vi "Sub00_Setup.vi"(7 "Enum":T1(ring), 8 "error in (no error)":errorcluster, 9 "Tab Control":T2(tab), 10 "Select sequence":string(combo)="F1", 11 "Path":path) -> (0 "error out":errorcluster, 1 "filenames":string[](array[string]), 2 "name":string, 3 "path out":path)   [LabVIEW 2019]
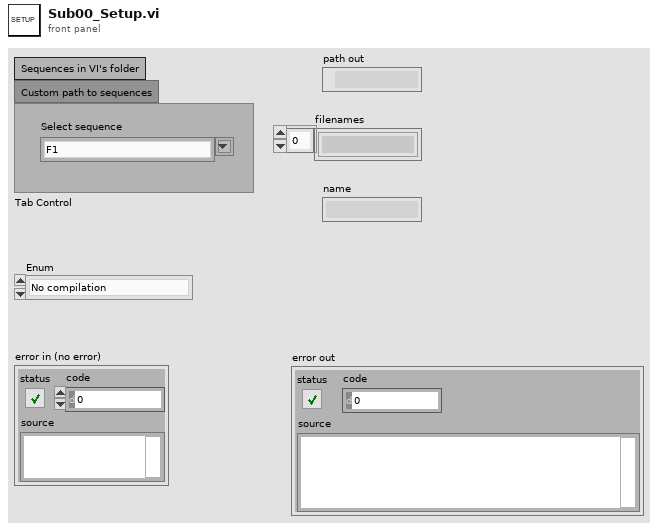
[diagram p1: front panel]
types:
  T1 = enum16{"No compilation", "No memory", "With memory", "Simple"}
  T2 = enum32{"Sequences in VI's folder", "Custom path to sequences"}
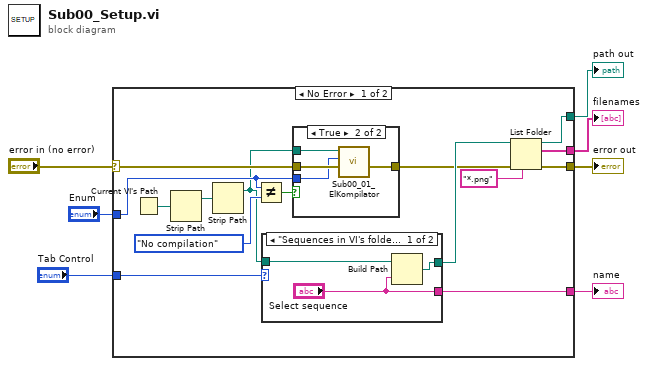
[diagram p0: block diagram]
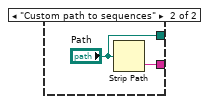
[diagram p3: hidden frame]
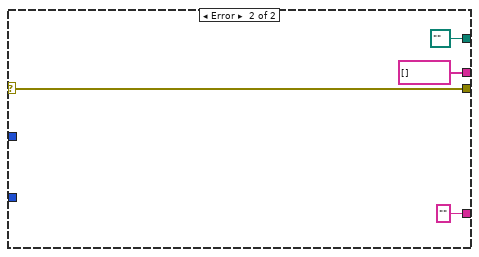
[diagram p4: hidden frame]
diagram:
  n1 = case shown="No Error" "error in (no error)" {
    selector: "error in (no error)" -> [w15 w33]
    tunnel: [w21 w33] -> w7
    tunnel: [w20 path "" ("path out")] -> w6
    tunnel: [w19 string[] [] ("filenames")] -> w5
    tunnel: [w17 "" ("name")] -> w4
    tunnel: "Enum" -> [w13 _]
    tunnel: "Tab Control" -> [w16 _]
    frame No Error {
      n2 = Current VI's Path() -> (path=w9:path)
      n3 = Strip Path(path=w9) -> (stripped path=w10:path)  [unwired: 1 out]
      n4 = Strip Path(path=w10) -> (stripped path=w8:path)  [unwired: 1 out]
      n5 = Not Equal?(x=w13, y=T1."No compilation") -> (x != y?=w11:bool)
      n6 = case shown="\"Sequences in VI's folder\", Default" w16 {
        tunnel: ["Select sequence" w31] -> w17
        tunnel: w8 -> [w29 _]
        tunnel: [w28 "Path"] -> w22
        frame "Sequences in VI's folder", Default {
          n7 = Build Path(base path=w29, name or relative path="Select sequence") -> (appended path=w28:path)
        }
        frame "Custom path to sequences" {
          n8 = Strip Path(path="Path") -> (name=w31:string)  [unwired: 1 out]
        }
      }
      n9 = case shown="True" w11 {
        tunnel: w15 -> [w23 w26]
        tunnel: w13 -> [_ w25]
        tunnel: [w23 w24] -> w12
        tunnel: w8 -> [_ w27]
        frame False {
        }
        frame True {
          n10 = call "Sub00_01_ElKompilator.vi"("error in (no error)"=w26, "Enum"=w25, "base path"=w27) -> ("error out"=w24:errorcluster)  [unwired: 8 in]
        }
      }
      n11 = List Folder(path=w22, pattern="*.png", error in=w12) -> (path out=w20:path, filenames=w19:string[], error out=w21:errorcluster)  [unwired: 1 in, 1 out]
    }
    frame Error {
    }
  }
  "error out" <- w7
  "path out" <- w6
  "filenames" <- w5
  "name" <- w4
